vi "ArmGrabberMastControl.vi"(8 "error in (no error)":errorcluster, 11 "Robot Commands":T1) -> (0 "error out":errorcluster)   [LabVIEW 2014]
uses:
  Joystick/Robot Commands.ctl
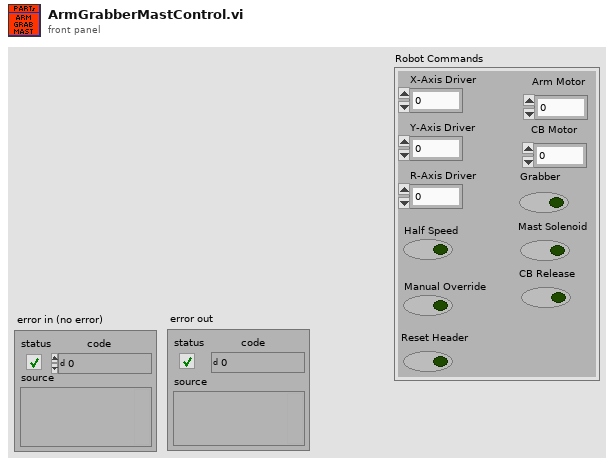
[diagram p1: front panel]
types:
  T1 = typedef "Robot Commands.ctl" = cluster{"X-Axis Driver":dbl, "Y-Axis Driver":dbl, "R-Axis Driver":dbl, "Half Speed":bool, "Manual Override":bool, "Reset Header":bool, "Arm Motor":dbl, "CB Motor":dbl, "Grabber":bool, "Mast Solenoid":bool, "CB Release":bool}
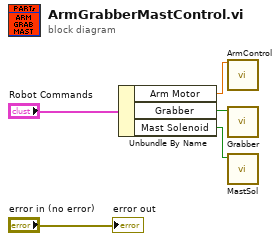
[diagram p0: block diagram]
diagram:
  n1 = Unbundle By Name("Robot Commands") -> ("Arm Motor"=w3:dbl, "Grabber"=w2:bool, "Mast Solenoid"=w1:bool)
  n2 = call "ArmControl.vi"("Arm Value"=w3) -> ()  [unwired: 14 in, 1 out]
  n3 = call "Grabber.vi"("Grabber Open/Close"=w2) -> ()  [unwired: 10 in, 1 out]
  n4 = call "MastSol.vi"("Piston U/D"=w1) -> ()  [unwired: 10 in, 1 out]
  "error out" <- "error in (no error)"
